vi "Show Settings UI.vi"(8 "Error In":errorcluster, 11 "Splitter in":refnum<class "Splitter.lvclass">) -> (0 "Error Out":errorcluster, 3 "Splitter out":refnum<class "Splitter.lvclass">)   [LabVIEW 2017, in "Splitter.lvclass"]
uses:
  Splitter.lvclass
  D:/software/LabView_PaneRelief_2017/test/D/software/LabView_PaneRelief_2017/Classes/Panel Object/Panel Object.lvclass
  Panel Object/Panel Object.lvclass/Panel Object.ctl
  Splitter Settings UI/Splitter Settings UI Messages/Show Splitter Settings UI Msg/Show Splitter Settings UI Msg.lvclass/Show Splitter Settings UI Msg.ctl
  <vilib>/ActorFramework/Message Enqueuer/Message Enqueuer.lvclass/Message Enqueuer.ctl
  Panel Object/Read Settings UI Enqueuer.vi
  <vilib>/ActorFramework/Message Enqueuer/Enqueue.vi
  Splitter Settings UI/Splitter Settings UI Messages/Show Splitter Settings UI Msg/Show Splitter Settings UI Msg.lvclass
  C:/Program Files (x86)/National Instruments/LabVIEW 2017/vi.lib/ActorFramework/Message/Message.lvclass
  <vilib>/ActorFramework/Message Priority Queue/Priority Enqueue.vi
  <vilib>/ActorFramework/Message Enqueuer/Message Enqueuer.lvclass
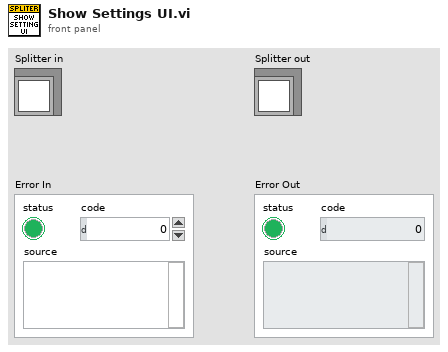
[diagram p1: front panel]
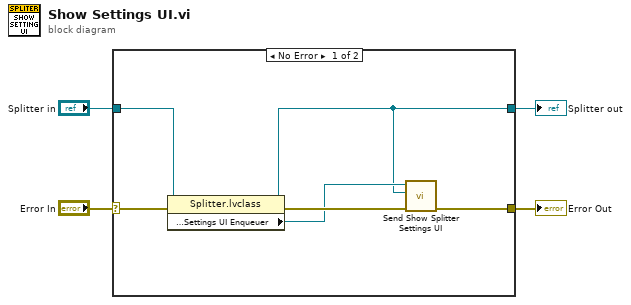
[diagram p0: block diagram]
diagram:
  n1 = case shown="No Error" "Error In" {
    selector: "Error In" -> [w10 w12]
    tunnel: [w7 w12] -> w1
    tunnel: [w5 w11] -> w3
    tunnel: "Splitter in" -> [w9 w11]
    frame No Error {
      n2 = property class="Splitter.lvclass"(reference=w9, error in=w10) -> (reference out=w5:refnum<class "Splitter.lvclass">, error out=w8:errorcluster, "Protected Accessors:Settings UI Enqueuer"=w6:refnum<class "Message Enqueuer.lvclass">)
      n3 = call "Send Show Splitter Settings UI.vi"("error in (no error)"=w8, "Splitter"=w5, "Message Enqueuer"=w6) -> ("error out"=w7:errorcluster)  [unwired: 7 in, 1 out]
    }
    frame Error {
    }
  }
  "Splitter out" <- w3
  "Error Out" <- w1
